vi "CanopenSendMsgPack.vi"(0 "COSDOdataW":refnum<vi>, 1 "写入数据类型":refnum<vi>, 2 "操作：":enum16{"SDO快速读取请求", "SDO快速写入请求"}(ring), 5 "COSDOdataS":refnum<vi>, 7 "从站号：":u8 max=127, 9 "索引：":u16 format="0x%04x", 11 "子索引：":u8 format="0x%02x") -> (6 "发送数据帧信息输出":T1 {"ADLC" max=64; "AID" max=536870911}, 8 "字符串":string)   [LabVIEW 2016]
uses:
  Ctrl/CAN_FrameInfo.ctl
panel:
  in  "发送数据帧信息输入":T1 {"ADLC" max=64; "AID" max=536870911}
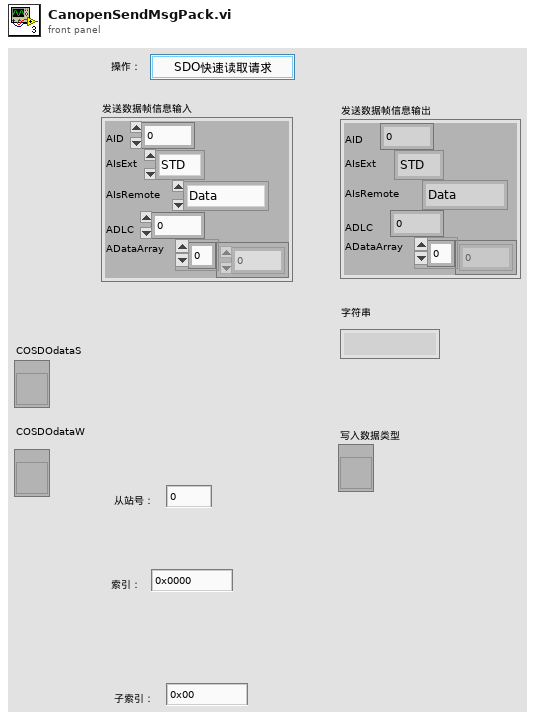
[diagram p1: front panel]
types:
  T1 = typedef "CAN_FrameInfo.ctl" = cluster{"AID":u32, "AIsExt":enum16{"STD", "EXT"}, "AIsRemote":enum16{"Data", "Remote"}, "ADLC":u8, "ADataArray":u8[]}
  T2 = enum16{"int8", "uint8", "int16", "uint16", "int32", "uint32"}
  T3 = enum8{"Enabled", "Disabled", "Disabled and Grayed Out"}
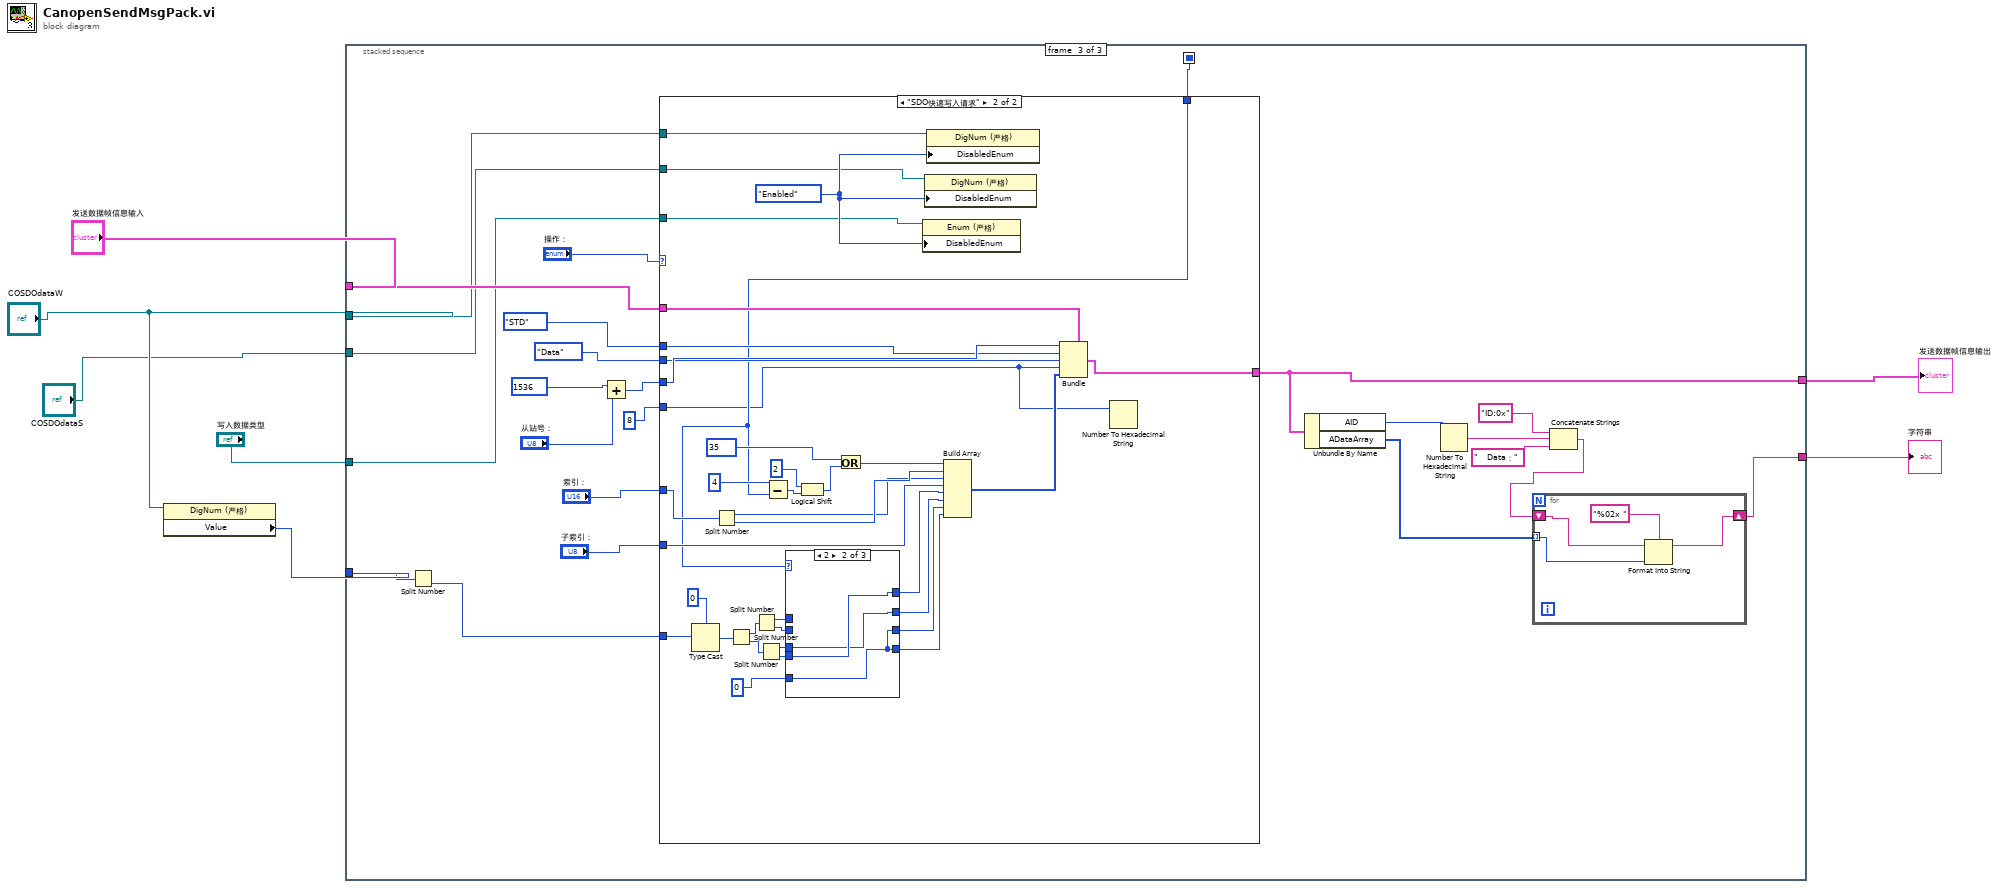
[diagram p0: block diagram]
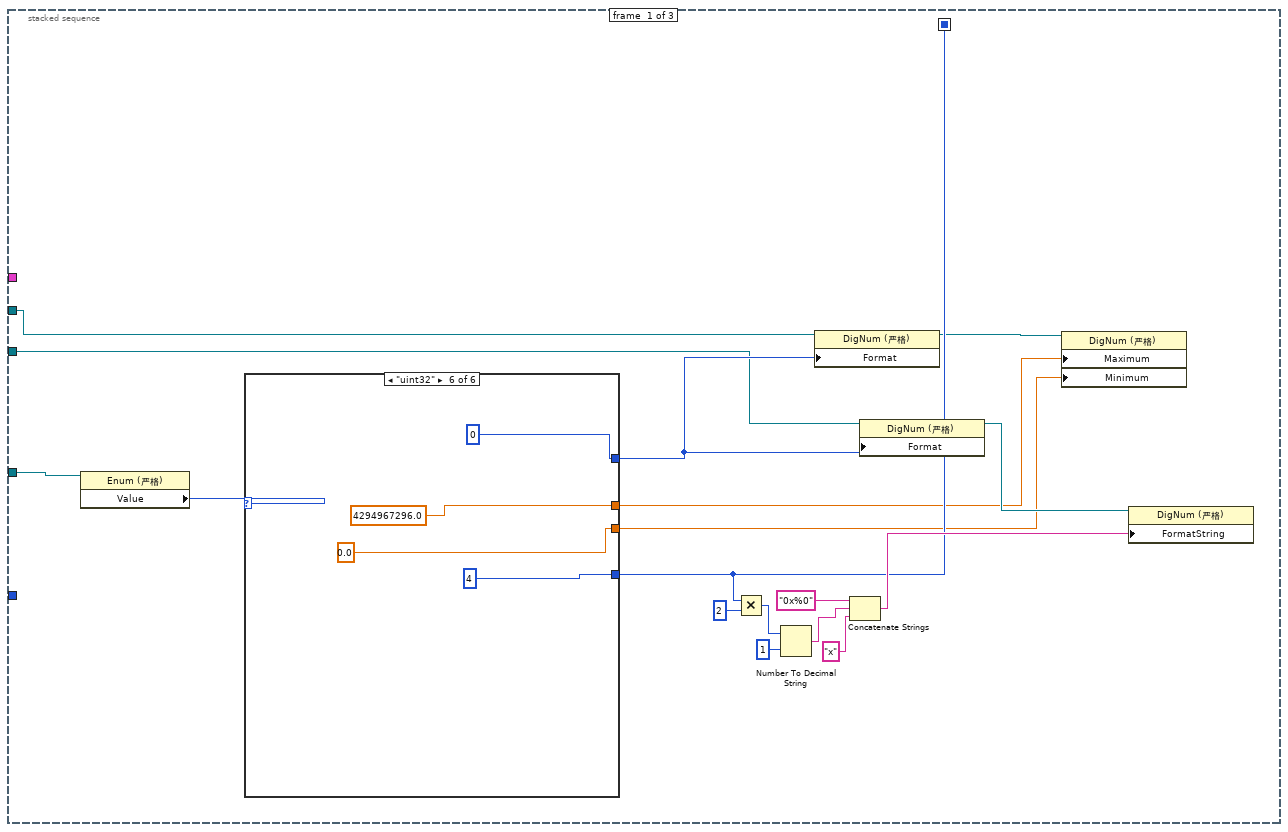
[diagram p2: hidden frame]
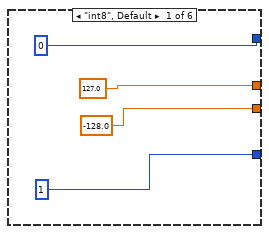
[diagram p3: hidden frame]
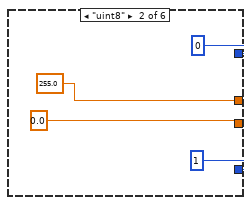
[diagram p4: hidden frame]
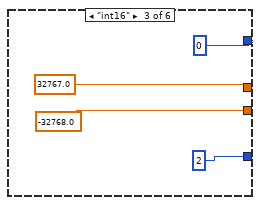
[diagram p5: hidden frame]
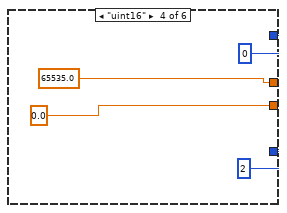
[diagram p6: hidden frame]
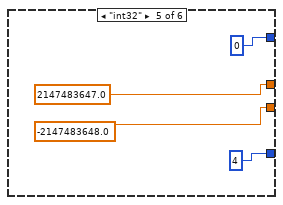
[diagram p7: hidden frame]
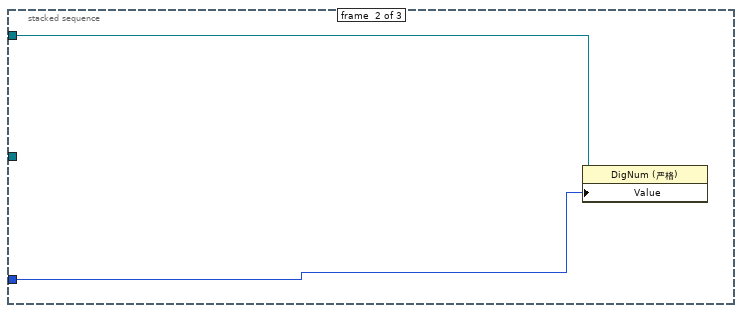
[diagram p8: hidden frame]
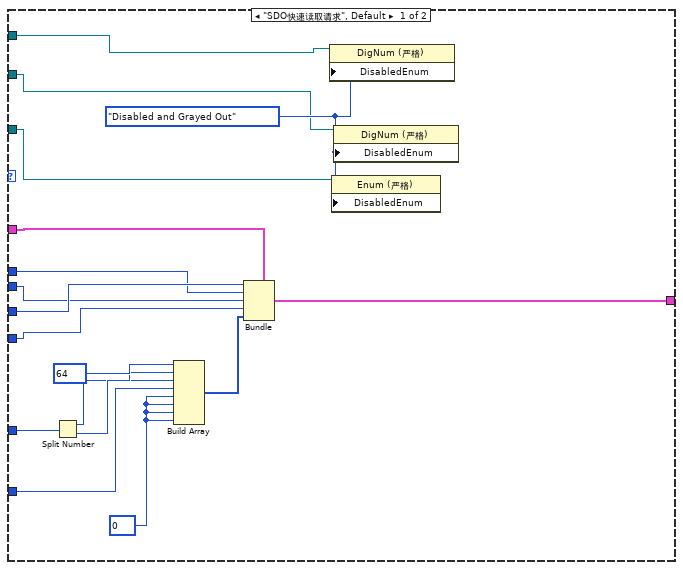
[diagram p9: hidden frame]
diagram:
  n1 = property class="DigNum (严格)"(reference="COSDOdataW") -> ("Value"=w3:i64)  [unwired: 1 in, 2 out]
  n2 = stacked-sequence {
    seq-local: [w16 _ _] -> [_ _ w65]
    tunnel: w3 -> [_ w50 w52]
    tunnel: "发送数据帧信息输入" -> [_ _ w64]
    tunnel: [_ _ w60] -> w7
    tunnel: "COSDOdataW" -> [w15 _ w63]
    tunnel: "COSDOdataS" -> [w14 w49 w62]
    tunnel: "写入数据类型" -> [w12 _ w61]
    tunnel: [_ _ w53] -> w4
    frame #0 {
      n3 = property class="Enum (严格)"(reference=w12) -> ("Value"=w11:T2)  [unwired: 1 in, 2 out]
      n4 = case shown="\"uint32\"" w11 {
        tunnel: [i8 0 ("显示格式:格式") u8 0 ("显示格式:格式") i16 0 ("显示格式:格式") u16 0 ("显示格式:格式") 0 ("显示格式:格式") u32 0 ("显示格式:格式")] -> w24
        tunnel: [u8 1 ("显示格式:格式") u8 1 ("显示格式:格式") u8 2 ("显示格式:格式") u8 2 ("显示格式:格式") u8 4 ("显示格式:格式") u8 4 ("显示格式:格式")] -> w16
        tunnel: [127.0 255.0 32767.0 65535.0 2147483647.0 4294967296.0] -> w9
        tunnel: [-128.0 0.0 -32768.0 0.0 -2147483648.0 0.0] -> w8
        frame "int8", Default {
        }
        frame "uint8" {
        }
        frame "int16" {
        }
        frame "uint16" {
        }
        frame "int32" {
        }
        frame "uint32" {
        }
      }
      n5 = Multiply(x=w16, y=u8 2) -> (x*y=w20:u8)
      n6 = Number To Decimal String(number=w20, width (-)=i16 1 ("宽度(-)")) -> (decimal integer string=w18:string)
      n7 = property on="属性节点" class="DigNum (严格)"(reference=w15, "Format"=w24) -> (reference out=w10:refnum<vi>)  [unwired: 1 in, 1 out]
      n8 = Concatenate Strings("0x%0" ("字符串"), w18, "x" ("字符串")) -> (w17:string)
      n9 = property on="属性节点" class="DigNum (严格)"(reference=w14, "Format"=w24) -> (reference out=w13:refnum<vi>)  [unwired: 1 in, 1 out]
      n10 = property class="DigNum (严格)"(reference=w10, "Maximum"=w9, "Minimum"=w8) -> ()  [unwired: 1 in, 2 out]
      n11 = property on="属性节点" class="DigNum (严格)"(reference=w13, "FormatString"=w17) -> ()  [unwired: 1 in, 2 out]
    }
    frame #1 {
      n12 = property class="DigNum (严格)"(reference=w49, "Value"=w50) -> ()  [unwired: 1 in, 2 out]
    }
    frame #2 {
      n13 = Split Number(x=w52) -> (lo(x)=w51:u32)  [unwired: 1 out]
      n14 = Add(x=u32 1536, y="从站号：") -> (x+y=w71:u32)
      n15 = case shown="\"SDO快速写入请求\"" "操作：" {
        tunnel: w71 -> [w94 w131]
        tunnel: w64 -> [w95 w130]
        tunnel: enum16{"STD", "EXT"}."STD" ("AIsExt") -> [w93 w129]
        tunnel: enum16{"Data", "Remote"}."Data" ("AIsRemote") -> [w92 w128]
        tunnel: u8 8 ("ADLC") -> [w91 w106]
        tunnel: "索引：" -> [w89 w120]
        tunnel: "子索引：" -> [w86 w117]
        tunnel: [w83 w116] -> w60
        tunnel: w65 -> [_ w115]
        tunnel: w51 -> [_ w101]
        tunnel: w62 -> [w80 w110]
        tunnel: w63 -> [w81 w109]
        tunnel: w61 -> [w79 w108]
        frame "SDO快速读取请求", Default {
          w85 = u8 0
          w82 = T3."Disabled and Grayed Out" ("禁用")
          n16 = Split Number(x=w89) -> (hi(x)=w87:u8, lo(x)=w88:u8)
          n17 = Build Array(u8 64, w88, w87, w86, w85, w85, w85, w85) -> (w84:u8[])
          n18 = Bundle(cluster=w95, "AID"=w94, "AIsExt"=w93, "AIsRemote"=w92, "ADLC"=w91, "ADataArray"=w84) -> (w83:T1)
          n19 = property on="属性节点" class="DigNum (严格)"(reference=w81, "DisabledEnum"=w82) -> ()  [unwired: 1 in, 2 out]
          n20 = property on="属性节点" class="Enum (严格)"(reference=w79, "DisabledEnum"=w82) -> ()  [unwired: 1 in, 2 out]
          n21 = property on="属性节点" class="DigNum (严格)"(reference=w80, "DisabledEnum"=w82) -> ()  [unwired: 1 in, 2 out]
        }
        frame "SDO快速写入请求" {
          w127 = T3."Enabled" ("禁用")
          n22 = Type Cast(type=u32 0, x=w101) -> (*(type *) &x=w105:u32)
          n23 = Split Number(x=w120) -> (hi(x)=w118:u8, lo(x)=w119:u8)
          n24 = Split Number(x=w105) -> (hi(x)=w104:u16, lo(x)=w103:u16)
          n25 = Split Number(x=w104) -> (hi(x)=w97:u8, lo(x)=w98:u8)
          n26 = Split Number(x=w103) -> (hi(x)=w99:u8, lo(x)=w100:u8)
          n27 = Subtract(x=u8 4, y=w115) -> (x-y=w124:u8)
          n28 = case shown="2" w115 {
            tunnel: [w133 w136 w140] -> w114
            tunnel: [w132 w135 w139] -> w113
            tunnel: [w132 w134 w138] -> w112
            tunnel: [w132 w134 w137] -> w111
            tunnel: w100 -> [w133 w136 w140]
            tunnel: w99 -> [_ w135 w139]
            tunnel: w98 -> [_ _ w138]
            tunnel: w97 -> [_ _ w137]
            tunnel: u8 0 -> [w132 w134 _]
            frame 1, Default {
            }
            frame 2 {
            }
            frame 4 {
            }
          }
          n29 = Logical Shift(y=u8 2, x=w124) -> (x << y=w122:u8)
          n30 = Or(x=u8 35, y=w122) -> (x .or. y?=w121:u8)
          n31 = property on="属性节点" class="Enum (严格)"(reference=w108, "DisabledEnum"=w127) -> ()  [unwired: 1 in, 2 out]
          n32 = property on="属性节点" class="DigNum (严格)"(reference=w110, "DisabledEnum"=w127) -> ()  [unwired: 1 in, 2 out]
          n33 = property on="属性节点" class="DigNum (严格)"(reference=w109, "DisabledEnum"=w127) -> ()  [unwired: 1 in, 2 out]
          n34 = Build Array(w121, w119, w118, w117, w114, w113, w112, w111) -> (w107:u8[])
          n35 = Bundle(cluster=w130, "AID"=w131, "AIsExt"=w129, "AIsRemote"=w128, "ADLC"=w106, "ADataArray"=w107) -> (w116:T1)
          n36 = Number To Hexadecimal String(2:w106) -> ()  [unwired: 1 in, 1 out]
        }
      }
      n37 = Unbundle By Name(w60) -> ("AID"=w58:u32, "ADataArray"=w55:u8[])
      n38 = Number To Hexadecimal String(2:w58) -> (0:w57:string)  [unwired: 1 in]
      n39 = Concatenate Strings("ID:0x" ("字符串"), w57, "   Data：" ("字符串")) -> (w54:string)
      n40 = for {
        tunnel: w55 -> [w77] mode=indexing
        shift-right: [w76] -> w53
        shift-left: w54 -> [w75]
        n41 = Format Into String(format string="%02x " ("格式字符串"), initial string=w75, w77) -> (resulting string=w76:string)  [unwired: 1 in, 1 out]
      }
    }
  }
  "字符串" <- w4
  "发送数据帧信息输出" <- w7
